vi "InsightCMConsoleExe.vi"(5 "definitionTypes":T1(ring), 7 "method":T2(ring), 10 "ExportDirectoryPath":path=path "E:/ExportedDefinitions", 11 "TrunkPath":path=path "E:/development/NICM/Source/R2/Trunk/Binaries/Debug") -> (0 "error out":errorcluster, 3 "String":string)   [LabVIEW 2017]
panel:
  out "cmd line":string
  in  "definitionTypeName":string
  in  "NewName":string
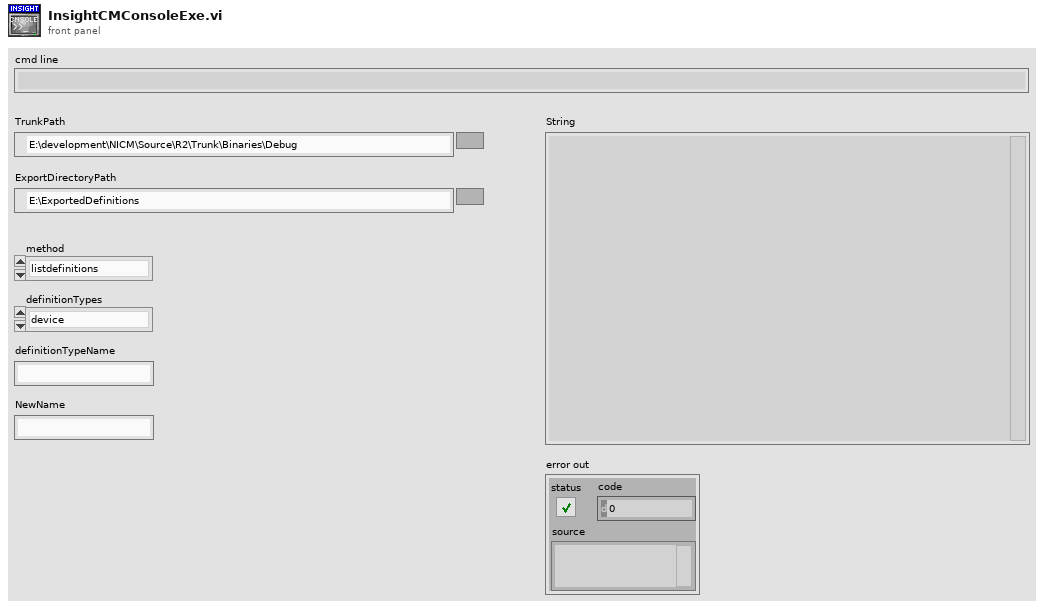
[diagram p1: front panel]
types:
  T1 = enum16{"device", "module", "channel", "metric", "instance", "unit"}
  T2 = enum16{"listdefinitions", "exportdefinition", "importdefinition", "deletedefinition"}
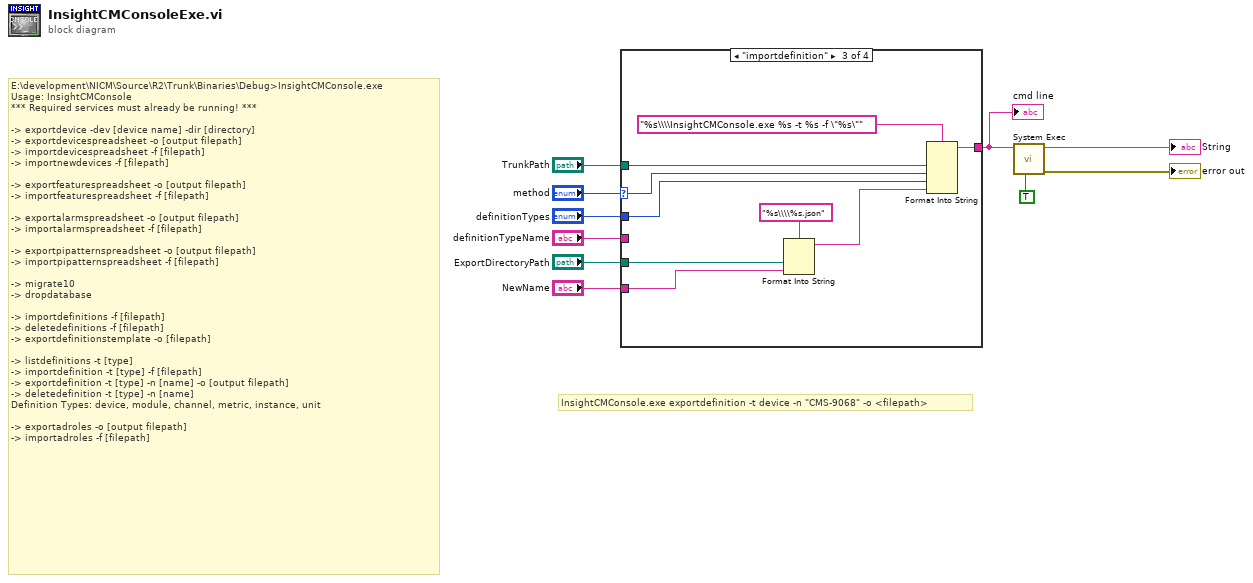
[diagram p0: block diagram]
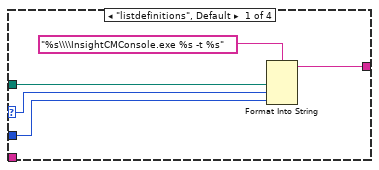
[diagram p2: hidden frame]
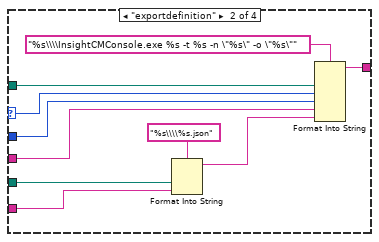
[diagram p3: hidden frame]
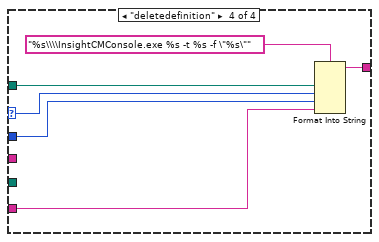
[diagram p4: hidden frame]
diagram:
  # "InsightCMConsole.exe exportdefinition -t device -n \"CMS-9068\" -o <filepath>"
  # "E:\\development\\NICM\\Source\\R2\\Trunk\\Binaries\\Debug>InsightCMConsole.exe\nUsage: InsightCMConsole\n*** Required services must already be running! ***\n\n-> exportdevice -dev [device name] -dir [directory]\n-> exportdevicespreadsheet -o [output filepath]\n-> importdevicespreadsheet -f [filepath]\n-> importnewdevices -f [filepath]\n\n-> exportfeaturespreadsheet -o [output filepath]\n-> importfeaturespreadsheet -f [filepath]\n\n-> exportalarmspreadsheet -o [output filepath]\n-> importalarmspreadsheet -f [filepath]\n\n-> exportpipatternspreadsheet -o [output filepath]\n-> importpipatternspreadsheet -f [filepath]\n\n-> migrate10\n-> dropdatabase\n\n-> importdefinitions -f [filepath]\n-> deletedefinitions -f [filepath]\n-> exportdefinitionstemplate -o [filepath]\n\n-> listdefinitions -t [type]\n-> importdefinition -t [type] -f [filepath]\n-> exportdefinition -t [type] -n [name] -o [output filepath]\n-> deletedefinition -t [type] -n [name]\nDefinition Types: device, module, channel, metric, instance, unit\n\n-> exportadroles -o [output filepath]\n-> importadroles -f [filepath]"
  n1 = case shown="\"importdefinition\"" "method" {
    selector: "method" -> [w11 w21 w30 w36]
    tunnel: "TrunkPath" -> [w14 w24 w33 w39]
    tunnel: "definitionTypes" -> [w13 w23 w32 w38]
    tunnel: [w12 w22 w31 w37] -> w5
    tunnel: "NewName" -> [_ w18 w27 w35]
    tunnel: "ExportDirectoryPath" -> [_ w19 w28 _]
    tunnel: "definitionTypeName" -> [_ w16 _ _]
    frame "listdefinitions", Default {
      n2 = Format Into String(format string="%s\\\\InsightCMConsole.exe %s -t %s", w14, w11, w13) -> (resulting string=w12:string)  [unwired: 2 in, 1 out]
    }
    frame "exportdefinition" {
      n3 = Format Into String(format string="%s\\\\%s.json", w19, w18) -> (resulting string=w17:string)  [unwired: 2 in, 1 out]
      n4 = Format Into String(format string="%s\\\\InsightCMConsole.exe %s -t %s -n \"%s\" -o \"%s\"", w24, w21, w23, w16, w17) -> (resulting string=w22:string)  [unwired: 2 in, 1 out]
    }
    frame "importdefinition" {
      n5 = Format Into String(format string="%s\\\\%s.json", w28, w27) -> (resulting string=w26:string)  [unwired: 2 in, 1 out]
      n6 = Format Into String(format string="%s\\\\InsightCMConsole.exe %s -t %s -f \"%s\"", w33, w30, w32, w26) -> (resulting string=w31:string)  [unwired: 2 in, 1 out]
    }
    frame "deletedefinition" {
      n7 = Format Into String(format string="%s\\\\InsightCMConsole.exe %s -t %s -f \"%s\"", w39, w36, w38, w35) -> (resulting string=w37:string)  [unwired: 2 in, 1 out]
    }
  }
  "cmd line" <- w5
  n8 = call <vilib>:"System Exec.vi"("run minimized? (F)"=TRUE, "command line"=w5) -> ("error out"=→"error out":errorcluster, "standard output"=→"String":string)  [unwired: 6 in, 2 out]
